vi "PID Parameter Manager (DBL Array).vi"(0 "previous PID gains":T1(array[cluster]), 1 "PID gains":T1(array[cluster]), 3 "process variable size":i32, 5 "previous Kp":dbl[](array[numeric]), 7 "previous Ki":dbl[](array[numeric]), 9 "previous Kd":dbl[](array[numeric]), 11 "previous PID Gains equal ?":bool[](array[boolean]), 12 "initialize":bool) -> (4 "PID Parameter Out":T1(array[cluster]), 6 "Kp":dbl[](array[numeric]), 8 "Ki":dbl[](array[numeric]), 10 "Kd":dbl[](array[numeric]), 14 "all PID Gains equal ?":bool, 15 "PID Gains equal ?":bool[](array[boolean]))   [LabVIEW 2020, in "NI_PID_pid.lvlib"]
uses:
  <vilib>/addons/control/pid/NI_PID_pid.lvlib
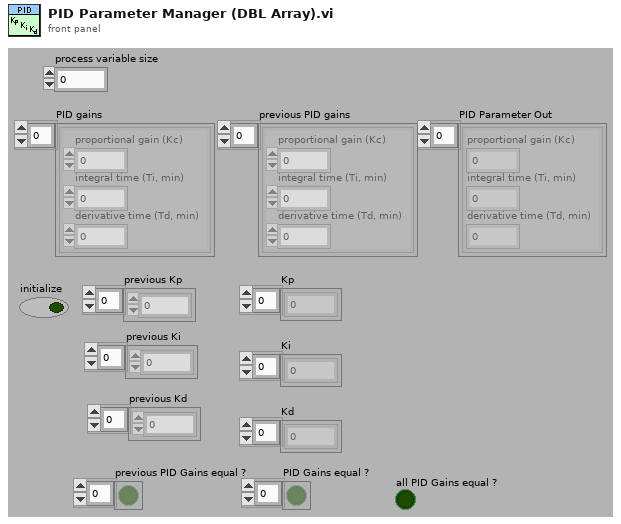
[diagram p1: front panel]
types:
  T1 = cluster{"proportional gain (Kc)":dbl, "integral time (Ti, min)":dbl, "derivative time (Td, min)":dbl}[]
  T2 = cluster{"proportional gain (Kc)":dbl, "integral time (Ti, min)":dbl, "derivative time (Td, min)":dbl}
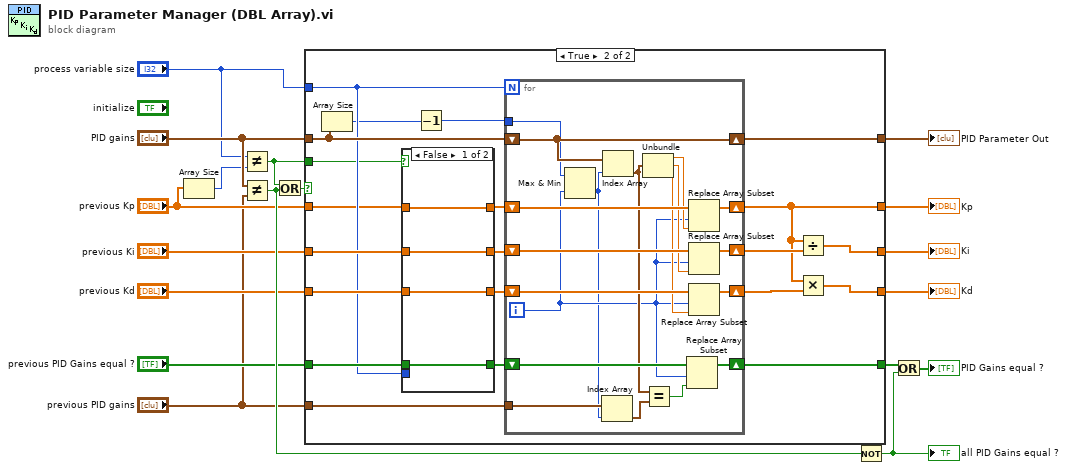
[diagram p0: block diagram]
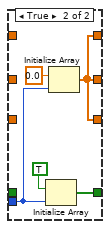
[diagram p3: hidden frame]
diagram:
  n1 = Array Size(array="previous Kp") -> (size(s)=w4:i32)
  n2 = Not Equal?(x="process variable size", y=w4) -> (x != y?=w2:bool)
  n3 = Not Equal?(x="PID gains", y="previous PID gains") -> (x != y?=w15:bool)
  n4 = Or(x=w2, y=w15) -> (x .or. y?=w10:bool)
  n5 = case shown="True" w10 {
    tunnel: [w23 w29] -> w18
    tunnel: [w21 w31] -> w17
    tunnel: [w22 w30] -> w16
    tunnel: [w20 w44] -> w14
    tunnel: "previous PID gains" -> [w20 w39]
    tunnel: "previous Kd" -> [w21 w33]
    tunnel: "previous Ki" -> [w22 w35]
    tunnel: "previous Kp" -> [w23 w25]
    tunnel: "PID gains" -> [_ w43]
    tunnel: "process variable size" -> [_ w27]
    tunnel: [w19 w28] -> w7
    tunnel: "previous PID Gains equal ?" -> [w19 w34]
    tunnel: w2 -> [_ w24]
    frame False {
    }
    frame True {
      n6 = Array Size(array=w43) -> (size(s)=w26:i32)
      n7 = case shown="False" w24 {
        tunnel: [w48 w49] -> w36
        tunnel: w27 -> [_ w52]
        tunnel: [w46 w50] -> w40
        tunnel: [w47 w49] -> w38
        tunnel: [w45 w49] -> w37
        tunnel: w25 -> [w48 _]
        tunnel: w35 -> [w47 _]
        tunnel: w34 -> [w46 _]
        tunnel: w33 -> [w45 _]
        frame False {
        }
        frame True {
          n8 = Initialize Array(TRUE, w52) -> (w50:bool[])
          n9 = Initialize Array(0.0 ("element"), w52) -> (w49:dbl[])
        }
      }
      n10 = Decrement(x=w26) -> (x-1=w32:i32)
      n11 = for {
        N: w27 -> [_]
        shift-right: [w66] -> w29
        shift-left: w36 -> [w72]
        shift-right: [w65] -> w41
        shift-left: w38 -> [w70]
        shift-right: [w64] -> w42
        shift-left: w37 -> [w69]
        shift-right: [w63] -> w44
        shift-left: w43 -> [w63]
        shift-right: [w61] -> w28
        shift-left: w40 -> [w62]
        tunnel: w39 -> [w60]
        tunnel: w32 -> [w55]
        i -> [w56]
        n12 = Max & Min(x=w55, y=w56) -> (min(x,y)=w54:i32)  [unwired: 1 out]
        n13 = Index Array(array=w60, index=w54) -> (element=w59:T2)
        n14 = Index Array(array=w63, index=w54) -> (element=w58:T2)
        n15 = Unbundle(w58) -> ("proportional gain (Kc)"=w71:dbl, "integral time (Ti, min)"=w68:dbl, "derivative time (Td, min)"=w67:dbl)
        n16 = Equal?(x=w58, y=w59) -> (x = y?=w57:bool)
        n17 = Replace Array Subset(array=w62, new element=w57, index=w56) -> (w61:bool[])
        n18 = Replace Array Subset(array=w72, new element=w71, index=w56) -> (w66:dbl[])
        n19 = Replace Array Subset(array=w70, new element=w68, index=w56) -> (w65:dbl[])
        n20 = Replace Array Subset(array=w69, new element=w67, index=w56) -> (w64:dbl[])
      }
      n21 = Divide(x=w29, y=w41) -> (x/y=w30:dbl[])
      n22 = Multiply(x=w29, y=w42) -> (x*y=w31:dbl[])
    }
  }
  "Kp" <- w18
  "Kd" <- w17
  "Ki" <- w16
  "PID Parameter Out" <- w14
  n23 = Not(x=w15) -> (.not. x?=w6:bool)
  "all PID Gains equal ?" <- w6
  n24 = Or(x=w7, y=w6) -> (x .or. y?=→"PID Gains equal ?":bool[])
